vi "Auto read numbers XYZ when press start.vi"() -> ()   [LabVIEW 2016]
uses:
  Classes/Controllers/Motion/Copy of A3200 Folder/A3200.lvclass
  D:/INTT/V1/Classes/Controllers/Motion/Copy of Motion Folder/Motion.lvclass
  <vilib>/Utility/file.llb/Read Delimited Spreadsheet (DBL).vi
  Classes/Controllers/Motion/Copy of Motion Folder/Motion.lvclass
panel:
  out "XYZTheta Out":dbl[](array[numeric])
  in  "stop":bool
  in  "start":bool
  out "XYZTheta Out 2":dbl[](array[numeric])
  in  "file path":path
  out "first row":dbl[](array[numeric])
  out "all rows":dbl[][](array[numeric])
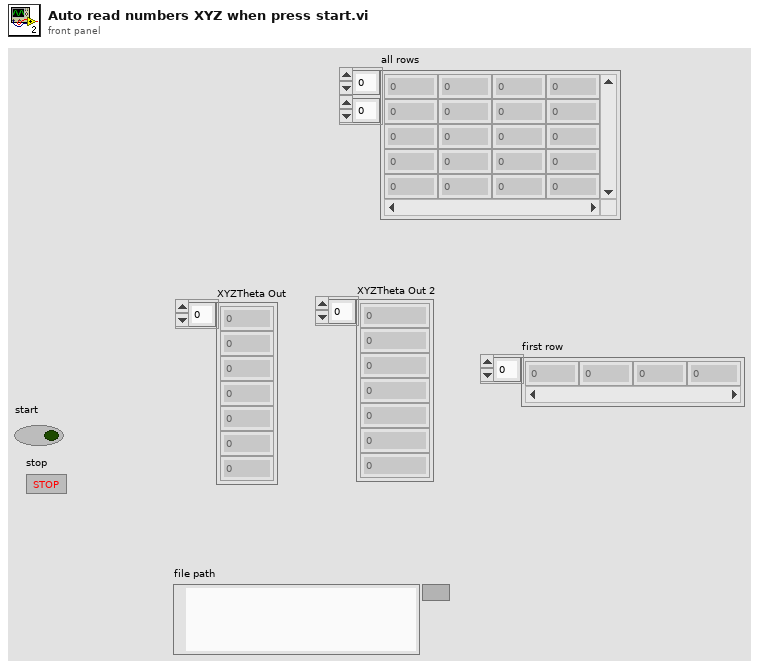
[diagram p1: front panel]
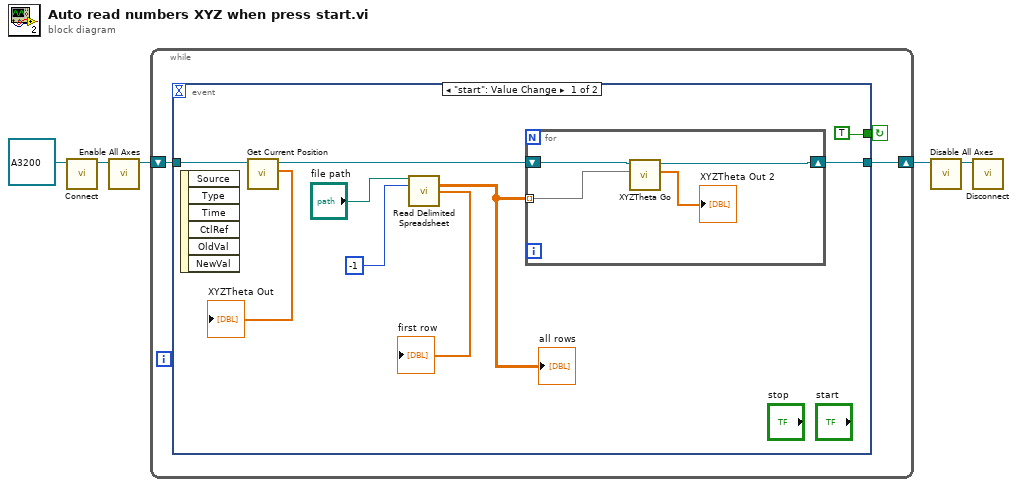
[diagram p0: block diagram]
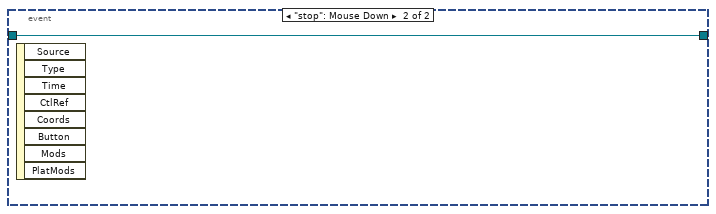
[diagram p2: hidden frame]
diagram:
  n1 = call-dynamic "Connect.vi"("Gantry in"=refnum<class "A3200.lvclass"> refnum ("Copy of A3200.lvclass")) -> ("Gantry out"=w4:refnum<class "A3200.lvclass">)  [unwired: 9 in, 1 out]
  n2 = call-dynamic "Enable All Axes.vi"("A3200 in"=w4) -> ("A3200 out"=w3:refnum<class "A3200.lvclass">)  [unwired: 9 in, 1 out]
  n3 = while {
    shift-right: [w8] -> w2
    shift-left: w3 -> [w7]
    stop <- w6 continue-if-true
    n4 = event shown="[0] \"start\": Value Change" {
      selector: _ -> [_ _]
      dyn-events: _ -> [_ _]
      timeout: _ -> [_ _]
      tunnel: [w17 w22] -> w8
      tunnel: w7 -> [w15 w22]
      tunnel: [TRUE _] -> w6
      event "start": Value Change {
        n5 = event-data() -> ()  [unwired: 1 in, 6 out]
        n6 = call-dynamic "Get Current Position.vi"("Gantry in"=w15) -> ("XYZTheta Out"=→"XYZTheta Out":dbl[], "Gantry out"=w14:refnum<class "A3200.lvclass">)  [unwired: 8 in, 1 out]
        n7 = call-poly <vilib>:"Read Delimited Spreadsheet.vi"("file path (dialog if empty)"="file path", "number of rows (all:-1)"=-1) -> ("all rows"=w9:dbl[][], "first row"=→"first row":dbl[])  [unwired: 8 in, 4 out]
        "all rows" <- w9
        n8 = for {
          shift-right: [w21] -> w17
          shift-left: w14 -> [w19]
          tunnel: w9 -> [w18] mode=indexing
          n9 = call "XYZTheta Go.vi"("XYZTheta In"=w18, "Motion in"=w19) -> ("XYZTheta Out"=→"XYZTheta Out 2":dbl[], "Motion out"=w21:refnum<class "A3200.lvclass">)  [unwired: 7 in, 1 out]
        }
      }
      event "stop": Mouse Down {
        n10 = event-data() -> ()  [unwired: 1 in, 8 out]
      }
    }
  }
  n11 = call-dynamic "Disable All Axes.vi"("Gantry in"=w2) -> ("Gantry out"=w1:refnum<class "A3200.lvclass">)  [unwired: 9 in, 1 out]
  n12 = call-dynamic "Disconnect.vi"("Gantry in"=w1) -> ()  [unwired: 9 in, 1 out]
